vi "Read Angel (rad) 2.vi"(11 "ValveModbus in":refnum<class "NeedleValve.lvclass">) -> (2 "Angel (rad)":dbl, 3 "ValveModbus out":refnum<class "NeedleValve.lvclass">)   [LabVIEW 2019, in "NeedleValve.lvclass"]
uses:
  NeedleValve.lvclass
  NeedleValve.lvclass/NeedleValve.ctl
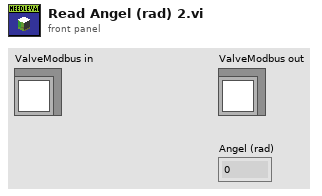
[diagram p1: front panel]
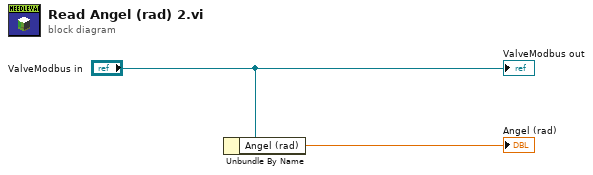
[diagram p0: block diagram]
diagram:
  n1 = Unbundle By Name("ValveModbus in") -> ("Angel (rad)"=→"Angel (rad)":dbl)
  "ValveModbus out" <- "ValveModbus in"
